vi "RSZVB Get Time Domain Transformation Type.vi"(8 "error in (no error)":errorcluster {"code" format="%.0x"}, 10 "Channel (Trace) (1)":i32=1, 11 "VISA session":refnum<visa-resource-name>) -> (0 "error out":errorcluster {"code" format="%.0x"}, 2 "Transformation Type":i32, 3 "dup VISA session":refnum<visa-resource-name>)   [LabVIEW 2011]
doc: "This VI queries the time domain transformation type.\n\nRemote-control command(s):\nCALCulate<Ch/Tr>:TRANsform:TIME[:TYPE]?\nCALCulate<Ch/Tr>:TRANsform:TIME:STIMulus?"
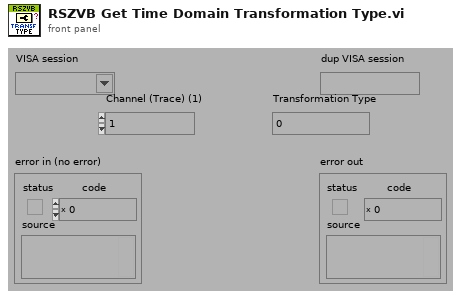
[diagram p1: front panel]
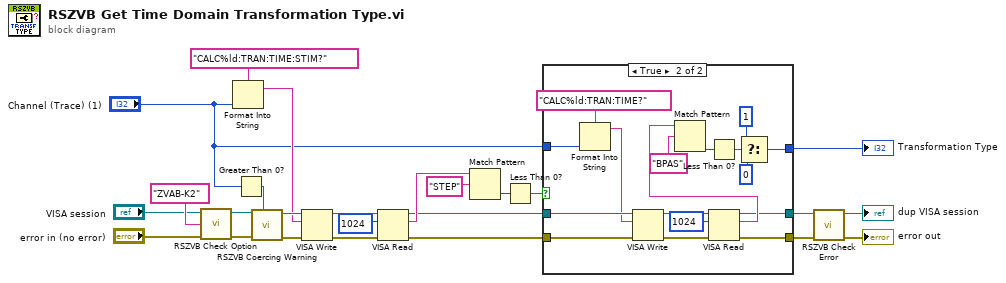
[diagram p0: block diagram]
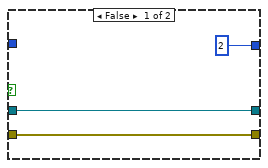
[diagram p2: hidden frame]
diagram:
  n1 = call "RSZVB Check Option.vi"("error in (no error)"="error in (no error)", "Options"="ZVAB-K2", "VISA session"="VISA session") -> ("error out"=w16:errorcluster, "dup VISA session"=w15:refnum<visa-resource-name>)  [unwired: 7 in]
  n2 = Format Into String(format string="CALC%ld:TRAN:TIME:STIM?", "Channel (Trace) (1)") -> (resulting string=w22:string)  [unwired: 2 in, 1 out]
  n3 = Greater Than 0?(x="Channel (Trace) (1)") -> (x > 0?=w18:bool)
  n4 = call "RSZVB Coercing Warning.vi"("In Range?"=w18, "error in (no error)"=w16, "VISA session"=w15) -> ("error out"=w23:errorcluster, "dup VISA session"=w24:refnum<visa-resource-name>)  [unwired: 7 in]
  n5 = VISA Write(VISA resource name=w24, write buffer=w22, error in (no error)=w23) -> (VISA resource name out=w20:refnum<visa-resource-name>, error out=w19:errorcluster)  [unwired: 1 out]
  n6 = VISA Read(VISA resource name=w20, byte count=u32 1024 ("byte count (0)"), error in (no error)=w19) -> (VISA resource name out=w4:refnum<visa-resource-name>, read buffer=w6:string, error out=w5:errorcluster)  [unwired: 1 out]
  n7 = Match Pattern(string=w6, regular expression="STEP") -> (offset past match=w10:i32)  [unwired: 1 in, 3 out]
  n8 = Less Than 0?(x=w10) -> (x < 0?=w8:bool)
  n9 = case shown="True" w8 {
    tunnel: [2 w40] -> w7
    tunnel: w5 -> [w27 w36]
    tunnel: w4 -> [w26 w35]
    tunnel: [w27 w33] -> w3
    tunnel: [w26 w32] -> w2
    tunnel: "Channel (Trace) (1)" -> [_ w31]
    frame False {
    }
    frame True {
      n10 = Format Into String(format string="CALC%ld:TRAN:TIME?", w31) -> (resulting string=w29:string)  [unwired: 2 in, 1 out]
      n11 = VISA Write(VISA resource name=w35, write buffer=w29, error in (no error)=w36) -> (VISA resource name out=w38:refnum<visa-resource-name>, error out=w37:errorcluster)  [unwired: 1 out]
      n12 = VISA Read(VISA resource name=w38, byte count=u32 1024 ("byte count (0)"), error in (no error)=w37) -> (VISA resource name out=w32:refnum<visa-resource-name>, read buffer=w34:string, error out=w33:errorcluster)  [unwired: 1 out]
      n13 = Match Pattern(string=w34, regular expression="BPAS") -> (offset past match=w44:i32)  [unwired: 1 in, 3 out]
      n14 = Less Than 0?(x=w44) -> (x < 0?=w43:bool)
      n15 = Select(t=1, s=w43, f=0) -> (s? t:f=w40:i32)
    }
  }
  "Transformation Type" <- w7
  n16 = call "RSZVB Check Error.vi"("error in (no error)"=w3, "VISA session"=w2) -> ("error out"=→"error out":errorcluster, "dup VISA session"=→"dup VISA session":refnum<visa-resource-name>)  [unwired: 8 in]
